vi "Init Settings Array.vi"(8 "error in (no error)":errorcluster, 11 "PRM in":refnum<class "PRM.lvclass">) -> (0 "error out":errorcluster, 3 "PRM out":refnum<class "PRM.lvclass">)   [LabVIEW 2019, in "PRM.lvlib" / "PRM.lvclass"]
uses:
  Library/PRM.lvclass
  Library/PRM.lvclass/PRM.ctl
  Custom Controls/RTD Parameters.ctl
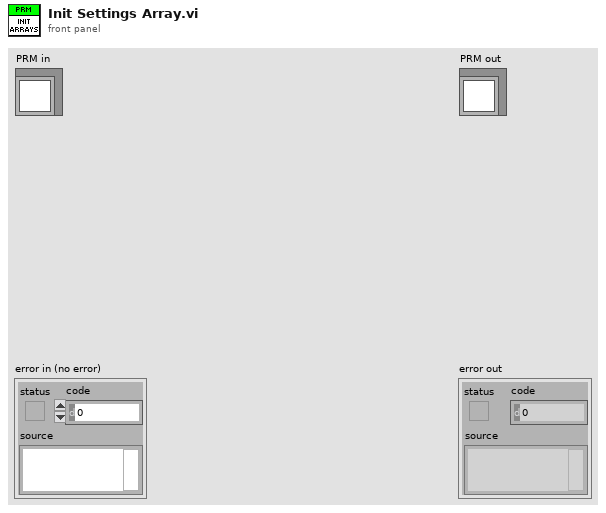
[diagram p1: front panel]
types:
  T1 = typedef "PRM.lvlib/PRM.lvclass/RTD Parameters.ctl" = cluster{"A":dbl, "B":dbl, "C":dbl, "R0":dbl}
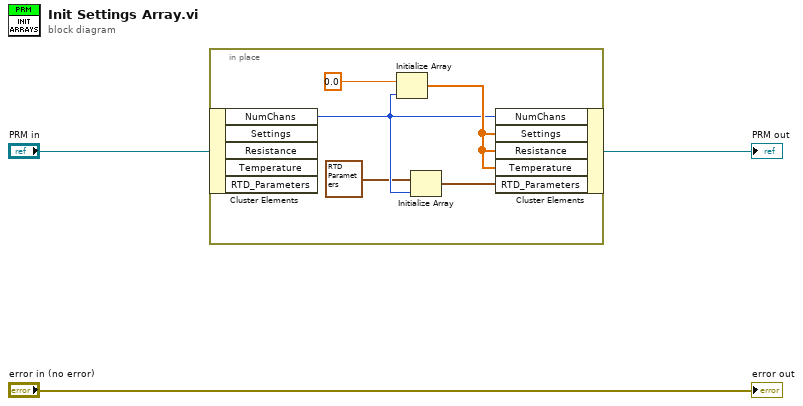
[diagram p0: block diagram]
diagram:
  n1 = in-place {
    n2 = in-place-cluster #1("PRM in") -> ("NumChans"=w6:i32)  [unwired: 4 out]
    n3 = Initialize Array(0.0, w6) -> (w7:dbl[])
    n4 = Initialize Array(T1 {"A"=0.003809999907389283, "B"=-6.020000000717118e-07, "C"=-5.999999976025183e-12, "R0"=1000.0} ("Callendar-Van Dusen RTD parameters"), w6) -> (w5:T1[])
    n5 = in-place-cluster #1("NumChans"=w6, "Settings"=w7, "Resistance"=w7, "Temperature"=w7, "RTD_Parameters"=w5) -> (→"PRM out":refnum<class "PRM.lvclass">)
  }
  "error out" <- "error in (no error)"
